vi "Varient_number_check.vi"(8 "error in":errorcluster, 11 "Varient No.":u16) -> (0 "error out":errorcluster, 1 "Batch Size":i32, 2 "Varient Number":i32, 3 "Varient Name":string)   [LabVIEW 2017]
uses:
  <vilib>/Utility/config.llb/Read Key (I32).vi
  <vilib>/Utility/config.llb/NI_LVConfig.lvlib
panel:
  # "Varient no. check"
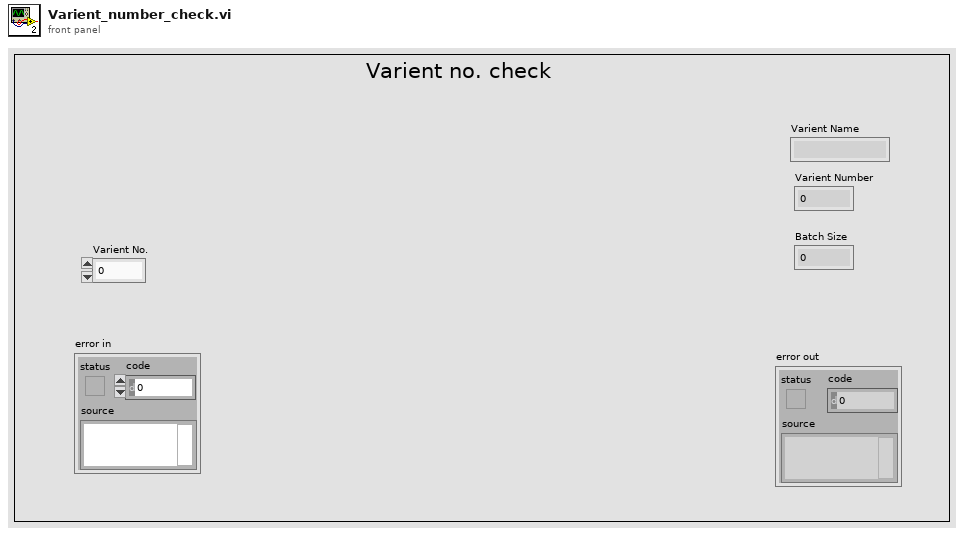
[diagram p1: front panel]
types:
  T1 = enum32{"invalid app kind", "Development System", "Run Time System", "Student Edition", "Embedded LabVIEW", "Evaluation", "Custom"}
  T2 = typedef "NI_LVConfig.lvlib/Config Data RefNum.ctl" = refnum<k1>
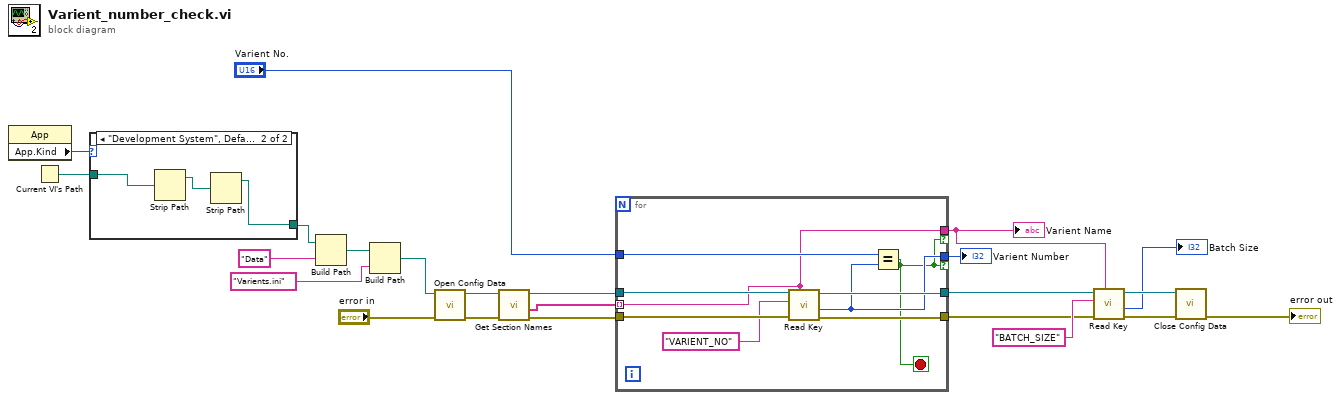
[diagram p0: block diagram]
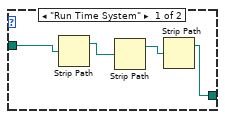
[diagram p2: hidden frame]
diagram:
  n1 = property class="App"() -> ("App.Kind"=w22:T1)  [unwired: 2 in, 2 out]
  n2 = Current VI's Path() -> (path=w23:path)
  n3 = case shown="\"Development System\", Default" w22 {
    tunnel: w23 -> [w25 w29]
    tunnel: [w24 w28] -> w20
    frame "Run Time System" {
      n4 = Strip Path(path=w25) -> (stripped path=w27:path)  [unwired: 1 out]
      n5 = Strip Path(path=w27) -> (stripped path=w26:path)  [unwired: 1 out]
      n6 = Strip Path(path=w26) -> (stripped path=w24:path)  [unwired: 1 out]
    }
    frame "Development System", Default {
      n7 = Strip Path(path=w29) -> (stripped path=w30:path)  [unwired: 1 out]
      n8 = Strip Path(path=w30) -> (stripped path=w28:path)  [unwired: 1 out]
    }
  }
  n9 = Build Path(base path=w20, name or relative path="Data") -> (appended path=w21:path)
  n10 = Build Path(base path=w21, name or relative path="Varients.ini") -> (appended path=w19:path)
  n11 = call <vilib>:"Open Config Data.vi"("error in (no error)"="error in", "configuration file path"=w19) -> ("error out"=w15:errorcluster, "refnum"=w16:T2)  [unwired: 7 in, 1 out]
  n12 = call <vilib>:"Get Section Names.vi"("error in (no error)"=w15, "refnum"=w16) -> ("error out"=w12:errorcluster, "section names"=w10:string[], "refnum out"=w11:T2)  [unwired: 7 in]
  n13 = for {
    tunnel: w10 -> [w32] mode=indexing
    tunnel: w11 -> [w37]
    tunnel: [w36] -> w4
    tunnel: w12 -> [w39]
    tunnel: [w38] -> w6
    tunnel: [w33] -> w8 if=w31
    tunnel: "Varient No." -> [w34]
    tunnel: [w32] -> w2 if=w31
    stop <- w31 stop-if-true
    n14 = call-poly <vilib>:"Read Key.vi"("section"=w32, "error in (no error)"=w39, "key"="VARIENT_NO" ("name or relative path"), "refnum"=w37) -> ("error out"=w38:errorcluster, "value"=w33:i32, "refnum out"=w36:T2)  [unwired: 4 in, 1 out]
    n15 = Equal?(x=w34, y=w33) -> (x = y?=w31:bool)
  }
  "Varient Number" <- w8
  "Varient Name" <- w2
  n16 = call-poly <vilib>:"Read Key.vi"("section"=w2, "error in (no error)"=w6, "key"="BATCH_SIZE" ("name or relative path"), "refnum"=w4) -> ("error out"=w5:errorcluster, "value"=→"Batch Size":i32, "refnum out"=w3:T2)  [unwired: 4 in, 1 out]
  n17 = call <vilib>:"Close Config Data.vi"("error in (no error)"=w5, "refnum"=w3) -> ("error out"=→"error out":errorcluster)  [unwired: 8 in, 1 out]
